vi "Write Object Name.vi"(8 "error in (no error)":errorcluster, 10 "Object Name":string, 11 "CS++Reference in":refnum<class "CS++Reference.lvclass">) -> (0 "error out":errorcluster, 3 "CS++Reference out":refnum<class "CS++Reference.lvclass">)   [LabVIEW 2012, in "CS++BaseClasses.lvlib" / "CS++Reference.lvclass"]
doc: "Write object name."
uses:
  CS++Reference.lvclass
  CS++Reference.lvclass/CS++Reference.ctl
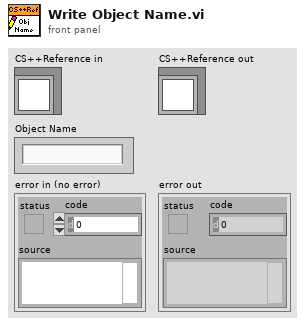
[diagram p1: front panel]
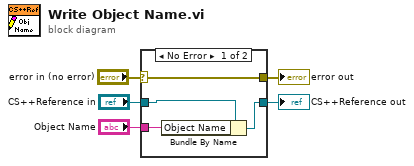
[diagram p0: block diagram]
diagram:
  n1 = case shown="No Error" "error in (no error)" {
    selector: "error in (no error)" -> [w9 w10]
    tunnel: [w9 w10] -> w4
    tunnel: [w7 w11] -> w2
    tunnel: "CS++Reference in" -> [w8 w11]
    tunnel: "Object Name" -> [w6 _]
    frame No Error {
      n2 = Bundle By Name(cluster=w8, "Object Name"=w6) -> (w7:refnum<class "CS++Reference.lvclass">)
    }
    frame Error {
    }
  }
  "error out" <- w4
  "CS++Reference out" <- w2
